vi "ENTRAINMENT VELOCITY_SSR TO MM_SEC CONVERSION.vi"(8 "error in (no error)":errorcluster, 10 "SSR":dbl, 11 "INITIAL Entrainment Speed":dbl) -> (0 "error out":errorcluster, 2 "Disc":dbl, 3 "Ball":dbl)   [LabVIEW 2025]
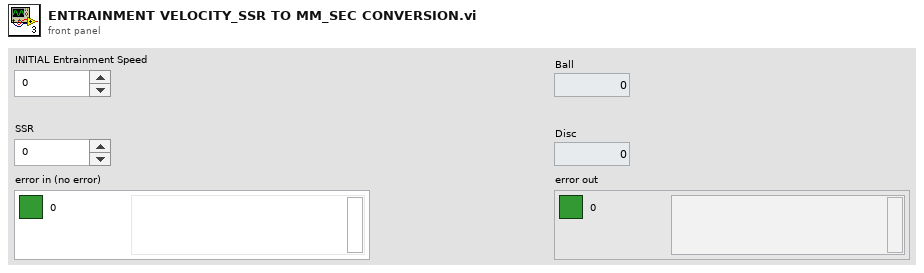
[diagram p1: front panel]
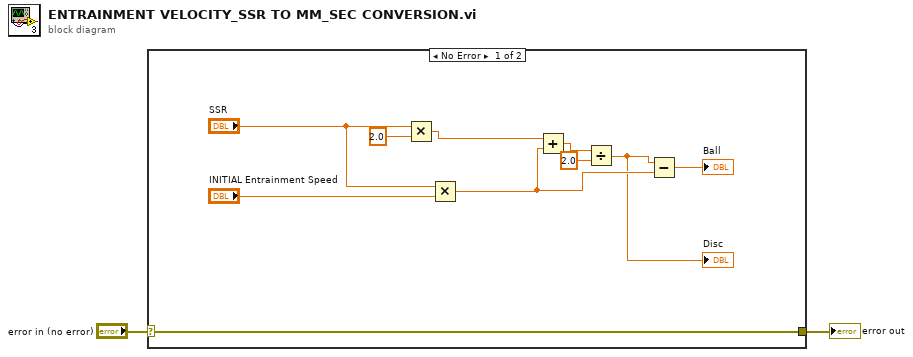
[diagram p0: block diagram]
diagram:
  n1 = case shown="No Error" "error in (no error)" {
    selector: "error in (no error)" -> [w3 _]
    tunnel: [w3 _] -> w1
    frame No Error {
      n2 = Multiply(x="SSR", y=2.0) -> (x*y=w9:dbl)
      n3 = Multiply(x="SSR", y="INITIAL Entrainment Speed") -> (x*y=w6:dbl)
      n4 = Add(x=w9, y=w6) -> (x+y=w8:dbl)
      n5 = Divide(x=w8, y=2.0) -> (x/y=w4:dbl)
      "Disc" <- w4
      n6 = Subtract(x=w4, y=w6) -> (x-y=→"Ball":dbl)
    }
    frame Error {
    }
  }
  "error out" <- w1
